vi "NewCluster.vi"(8 "R_th":i32=400, 9 "군집 원소 최수 개수":i32, 11 "x,y 배열":cluster{"x":dbl, "y":dbl}[](array[cluster])) -> (3 "클러스터링된 점 배열":cluster{cluster{"x":dbl, "y":dbl}[]}[](array[cluster]))   [LabVIEW 2015]
panel:
  out "배열":cluster{u32, dbl}[](array[cluster])
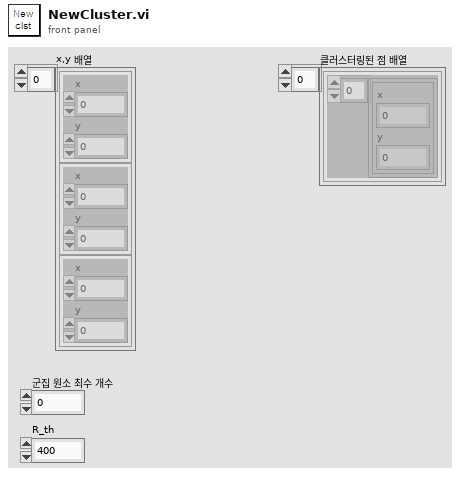
[diagram p1: front panel]
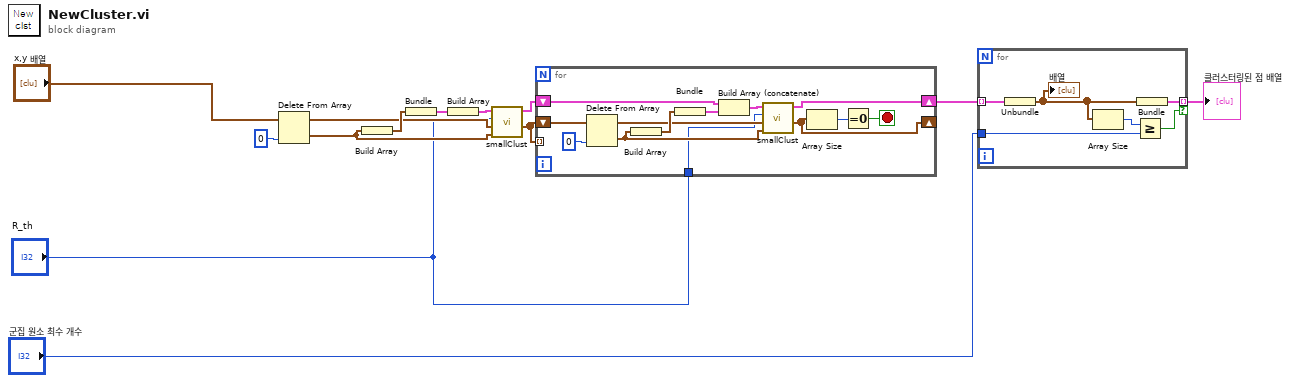
[diagram p0: block diagram]
diagram:
  n1 = Delete From Array(array="x,y 배열", index=0 ("인덱스")) -> (deleted portion=w7:cluster{"x":dbl, "y":dbl}, array with subset deleted=w6:cluster{"x":dbl, "y":dbl}[])  [unwired: 1 in]
  n2 = Build Array(w7) -> (w10:cluster{"x":dbl, "y":dbl}[])
  n3 = Bundle(w10) -> (w9:cluster{cluster{"x":dbl, "y":dbl}[]})  [unwired: 1 in]
  n4 = Build Array(w9) -> (w8:cluster{cluster{"x":dbl, "y":dbl}[]}[])
  n5 = call "smallClust.vi"("기준 원소"=w7, "미군집 원소"=w6, "R_th"="R_th", "미완성된 군집화"=w8) -> ("남은 미군집원소"=w4:cluster{"x":dbl, "y":dbl}[], "추가된 군집화"=w5:cluster{cluster{"x":dbl, "y":dbl}[]}[])  [unwired: 1 in, 1 out]
  n6 = for {
    tunnel: w4 -> [_] mode=indexing
    shift-right: [w17] -> _
    shift-left: w4 -> [w24]
    shift-right: [w18] -> w3
    shift-left: w5 -> [w21]
    tunnel: "R_th" -> [w14]
    stop <- w15 stop-if-true
    n7 = Delete From Array(array=w24, index=0 ("인덱스")) -> (deleted portion=w22:cluster{"x":dbl, "y":dbl}, array with subset deleted=w23:cluster{"x":dbl, "y":dbl}[])  [unwired: 1 in]
    n8 = Build Array(w22) -> (w25:cluster{"x":dbl, "y":dbl}[])
    n9 = Bundle(w25) -> (w20:cluster{cluster{"x":dbl, "y":dbl}[]})  [unwired: 1 in]
    n10 = Build Array (concatenate)(w21, w20) -> (w19:cluster{cluster{"x":dbl, "y":dbl}[]}[])
    n11 = call "smallClust.vi"("기준 원소"=w22, "미군집 원소"=w23, "R_th"=w14, "미완성된 군집화"=w19) -> ("남은 미군집원소"=w17:cluster{"x":dbl, "y":dbl}[], "추가된 군집화"=w18:cluster{cluster{"x":dbl, "y":dbl}[]}[])  [unwired: 1 in, 1 out]
    n12 = Array Size(array=w17) -> (size(s)=w16:i32)
    n13 = Equal To 0?(x=w16) -> (x = 0?=w15:bool)
  }
  n14 = for {
    tunnel: w3 -> [w32] mode=indexing
    tunnel: [w29] -> w2 mode=indexing if=w28
    tunnel: "군집 원소 최수 개수" -> [w27]
    n15 = Unbundle(w32) -> (w30:cluster{"x":dbl, "y":dbl}[])
    "배열" <- w30
    n16 = Array Size(array=w30) -> (size(s)=w31:i32)
    n17 = Greater Or Equal?(x=w31, y=w27) -> (x >= y?=w28:bool)
    n18 = Bundle(w30) -> (w29:cluster{cluster{"x":dbl, "y":dbl}[]})  [unwired: 1 in]
  }
  "클러스터링된 점 배열" <- w2
